vi "Sensor Till Stop.vi"() -> (3 "x .and. y?":bool)   [LabVIEW 2015]
uses:
  <vilib>/Rock Robotics/Network Tables/NT Read Boolean.vi
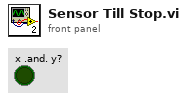
[diagram p1: front panel]
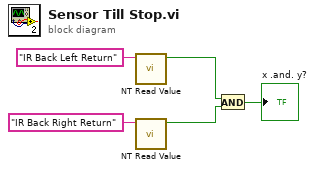
[diagram p0: block diagram]
diagram:
  n1 = call-poly <vilib>:"NT Read Value.vi"("Name"="IR Back Left Return") -> ("Boolean"=w4:bool)  [unwired: 9 in, 1 out]
  n2 = call-poly <vilib>:"NT Read Value.vi"("Name"="IR Back Right Return") -> ("Boolean"=w3:bool)  [unwired: 9 in, 1 out]
  n3 = And(x=w4, y=w3) -> (x .and. y?=→"x .and. y?":bool)
